vi "changeHWConfigChannel.vi"(8 "error in (no error)":errorcluster, 9 "state":string, 10 "channel":string, 11 "StaticOutputEditor in":refnum<class "StaticOutputEditor.lvclass">) -> (0 "error out":errorcluster, 3 "StaticOutputEditor out":refnum<class "StaticOutputEditor.lvclass">)   [LabVIEW 2011, in "Views.lvlib" / "ScriptEditor.lvlib" / "StaticOutputEditor.lvclass"]
uses:
  StaticOutputEditor.lvclass
  StaticOutputEditor.lvclass/StaticOutputEditor.ctl
  Tools/DatabaseHelpers/Database Objects/ChannelArray/ChannelArray.lvclass
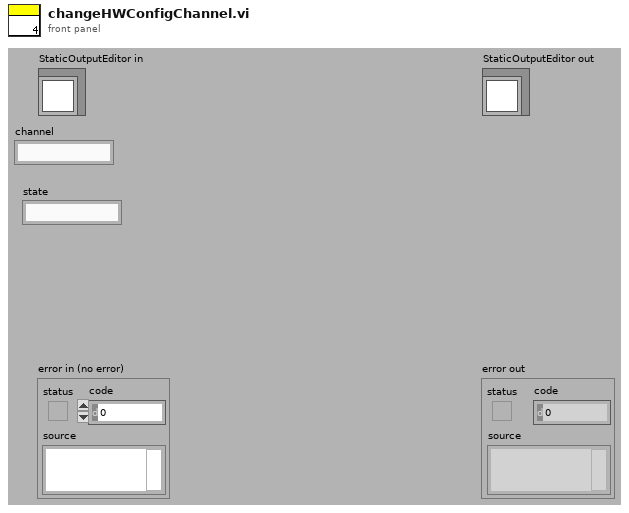
[diagram p1: front panel]
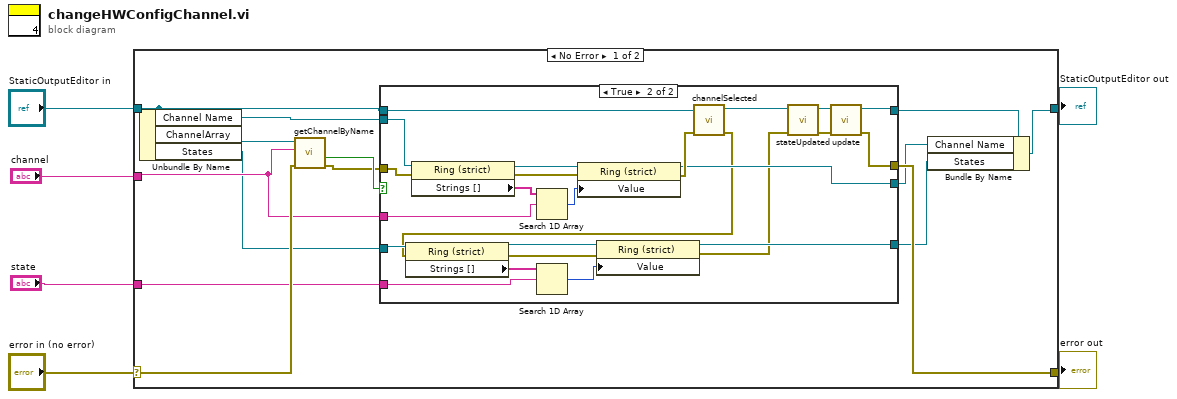
[diagram p0: block diagram]
diagram:
  n1 = case shown="No Error" "error in (no error)" {
    selector: "error in (no error)" -> [w19 w50]
    tunnel: [w11 w50] -> w5
    tunnel: [w7 w49] -> w3
    tunnel: "StaticOutputEditor in" -> [w17 w49]
    tunnel: "channel" -> [w15 _]
    tunnel: "state" -> [w13 _]
    frame No Error {
      n2 = Unbundle By Name(w17) -> ("Channel Name"=w16:refnum<vi>, "ChannelArray"=w20:refnum<class "ChannelArray.lvclass">, "States"=w14:refnum<vi>)
      n3 = call-dynamic "getChannelByName.vi"("error in (no error)"=w19, "channel_name"=w15, "ChannelArray in"=w20) -> ("error out"=w12:errorcluster, "found?"=w18:bool)  [unwired: 5 in, 2 out]
      n4 = case shown="True" w18 {
        tunnel: w17 -> [w24 w48]
        tunnel: [w24 w33] -> w8
        tunnel: w16 -> [w22 w47]
        tunnel: w12 -> [w23 w39]
        tunnel: w15 -> [_ w45]
        tunnel: w14 -> [w21 w40]
        tunnel: w13 -> [_ w37]
        tunnel: [w23 w32] -> w11
        tunnel: [w22 w31] -> w10
        tunnel: [w21 w30] -> w9
        frame False {
        }
        frame True {
          n5 = property class="Ring (strict)"(reference=w47, error in=w39) -> (reference out=w43:refnum<vi>, error out=w42:errorcluster, "Strings []"=w46:string[])
          n6 = Search 1D Array(1D array=w46, element=w45) -> (index of element=w41:i32)  [unwired: 1 in]
          n7 = property class="Ring (strict)"(reference=w43, error in=w42, "Value"=w41) -> (reference out=w31:refnum<vi>, error out=w44:errorcluster)
          n8 = call "channelSelected.vi"("error in (no error)"=w44, "StaticOutputEditor in"=w48) -> ("error out"=w29:errorcluster, "StaticOutputEditor out"=w28:refnum<class "StaticOutputEditor.lvclass">)  [unwired: 8 in]
          n9 = property class="Ring (strict)"(reference=w40, error in=w29) -> (reference out=w36:refnum<vi>, error out=w35:errorcluster, "Strings []"=w38:string[])
          n10 = Search 1D Array(1D array=w38, element=w37) -> (index of element=w34:i32)  [unwired: 1 in]
          n11 = property class="Ring (strict)"(reference=w36, error in=w35, "Value"=w34) -> (reference out=w30:refnum<vi>, error out=w26:errorcluster)
          n12 = call "stateUpdated.vi"("error in (no error)"=w26, "StaticOutputEditor in"=w28) -> ("error out"=w25:errorcluster, "StaticOutputEditor out"=w27:refnum<class "StaticOutputEditor.lvclass">)  [unwired: 8 in]
          n13 = call "update.vi"("error in (no error)"=w25, "StaticOutputEditor in"=w27) -> ("error out"=w32:errorcluster, "StaticOutputEditor out"=w33:refnum<class "StaticOutputEditor.lvclass">)  [unwired: 8 in]
        }
      }
      n14 = Bundle By Name(cluster=w8, "Channel Name"=w10, "States"=w9) -> (w7:refnum<class "StaticOutputEditor.lvclass">)
    }
    frame Error {
    }
  }
  "error out" <- w5
  "StaticOutputEditor out" <- w3
